vi "Test Complex Datatype.vi"(8 "error in (no error)":errorcluster) -> (0 "error out":errorcluster)   [LabVIEW 2018, in "JSON to LVConstant Test.lvlib"]
uses:
  JSON to LVConstant Test.lvlib
  <vilib>/addons/_JKI Toolkits/Caraya/classes/Test/Test.lvclass
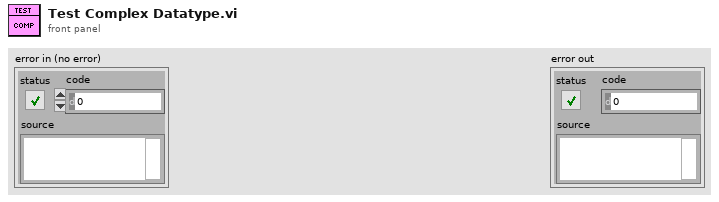
[diagram p1: front panel]
types:
  T1 = cluster{"Just String":string, "Just true":bool, "Just false":bool, "Just Number":i32, "Just String Array":string[], "Just true Array":bool[], "Just Number Array":i32[]}[]
  T2 = cluster{"Just String":string, "Just true":bool, "Just false":bool, "Just Number":i32, "Just String Array":string[], "Just true Array":bool[], "Just Number Array":i32[]}
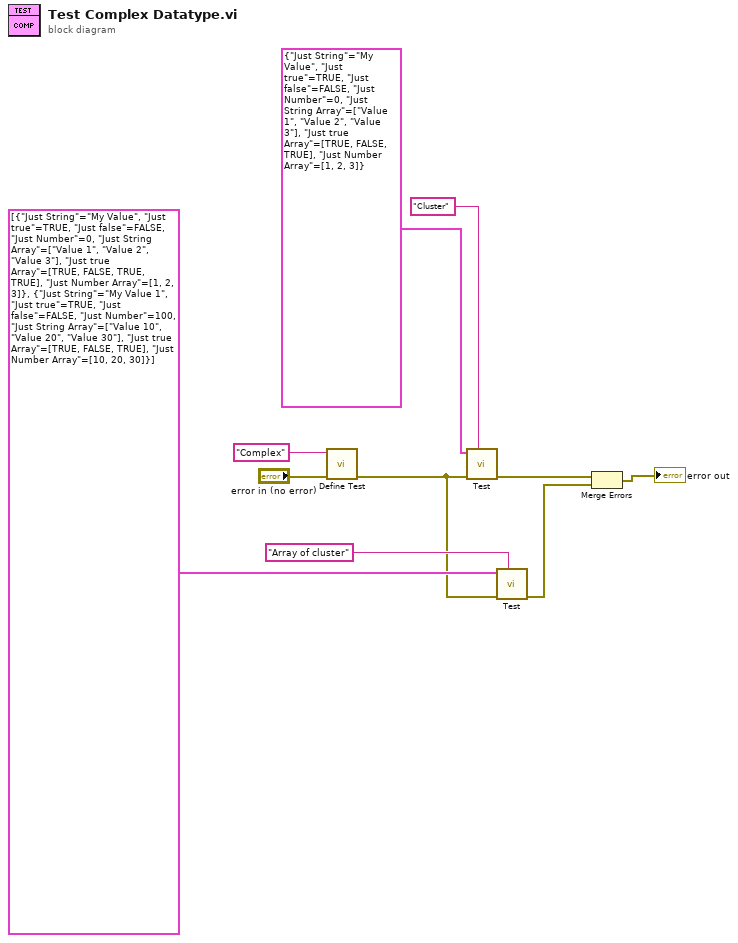
[diagram p0: block diagram]
diagram:
  n1 = call <vilib>:"Define Test.vi"("error in (no error)"="error in (no error)", "Label (VI Title)"="Complex") -> ("error out"=w2:errorcluster)  [unwired: 9 in]
  n2 = call "Test.vi"("Label (VI Title)"="Cluster", "error in (no error)"=w2, "Type"=T2 {"Just String"="My Value", "Just true"=TRUE, "Just false"=FALSE, "Just Number"=0, "Just String Array"=["Value 1", "Value 2", "Value 3"], "Just true Array"=[TRUE, FALSE, TRUE], "Just Number Array"=[1, 2, 3]}) -> ("error out"=w8:errorcluster)  [unwired: 8 in]
  n3 = call "Test.vi"("Label (VI Title)"="Array of cluster", "error in (no error)"=w2, "Type"=T1 [{"Just String"="My Value", "Just true"=TRUE, "Just false"=FALSE, "Just Number"=0, "Just String Array"=["Value 1", "Value 2", "Value 3"], "Just true Array"=[TRUE, FALSE, TRUE, TRUE], "Just Number Array"=[1, 2, 3]}, {"Just String"="My Value 1", "Just true"=TRUE, "Just false"=FALSE, "Just Number"=100, "Just String Array"=["Value 10", "Value 20", "Value 30"], "Just true Array"=[TRUE, FALSE, TRUE], "Just Number Array"=[10, 20, 30]}]) -> ("error out"=w3:errorcluster)  [unwired: 8 in]
  n4 = Merge Errors(w8, w3) -> (→"error out":errorcluster)
